vi "Add Calculate Channel_Formula_Formula.vi"(8 "error in (error out)":errorcluster, 9 "Formula Settings":T2, 10 "Calculated Channels Ref":refnum<k24>, 11 "SysDef Ref":T1) -> (0 "error out":errorcluster, 2 "Calculated Channels Ref Out":refnum<k24>)   [LabVIEW 2019, in "Simple SysDef API.lvlib"]
uses:
  <userlib>/SimpleSysDef/Simple SysDef API.lvlib
  NationalInstruments.VeriStand.SystemDefinitionAPI
  <userlib>/SimpleSysDef/_SubVIs/Add Calculate Channel_Formula_Settings.ctl
  <userlib>/SimpleSysDef/_SubVIs/System Definition Reference.ctl
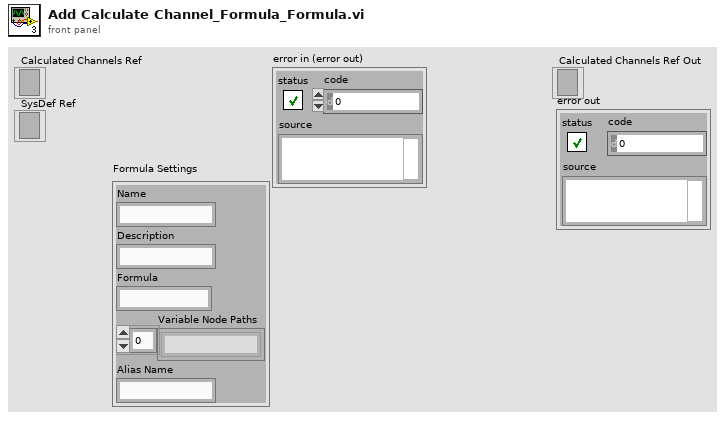
[diagram p1: front panel]
types:
  T1 = typedef "Simple SysDef API.lvlib/System Definition Reference.ctl" = refnum<k24>
  T2 = typedef "Simple SysDef API.lvlib/Add Calculate Channel_Formula_Settings.ctl" = cluster{"Name":string, "Description":string, "Formula":string, "Variable Node Paths":string[], "Alias Name":string}
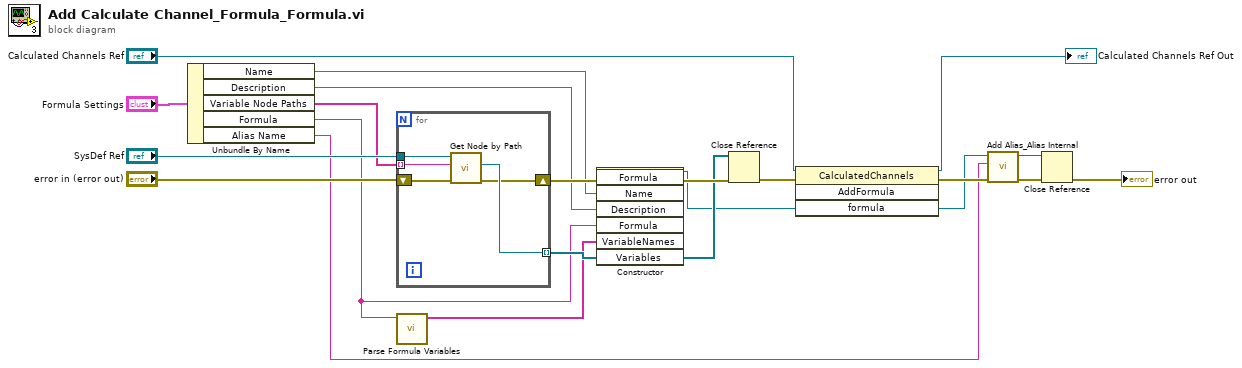
[diagram p0: block diagram]
diagram:
  n1 = Unbundle By Name("Formula Settings") -> ("Name"=w9:string, "Description"=w6:string, "Variable Node Paths"=w8:string[], "Formula"=w7:string, "Alias Name"=w1:string)
  n2 = for {
    tunnel: [w26] -> w15 mode=indexing
    shift-right: [w25] -> w11
    shift-left: "error in (error out)" -> [w24]
    tunnel: w8 -> [w23] mode=indexing
    tunnel: "SysDef Ref" -> [w22]
    n3 = call <userlib>:"Get Node by Path.vi"("error in (no error)"=w24, "System Definition Node Path"=w23, "SysDef Ref"=w22) -> ("error out"=w25:errorcluster, "Node Ref"=w26:refnum<k24>)  [unwired: 6 in, 1 out]
  }
  n4 = call <userlib>:"Parse Formula Variables.vi"("Formula"=w7) -> ("Variables"=w10:string[])  [unwired: 10 in]
  n5 = constructor class="Formula"(error in=w11, "Name"=w9, "Description"=w6, "Formula"=w7, "VariableNames"=w10, "Variables"=w15) -> (reference out=w3:refnum<k24>, error out=w14:errorcluster, "Variables"=w12:refnum<k24>[])  [unwired: 2 in, 5 out]
  n6 = Close Reference(reference=w12, error in (no error)=w14) -> (error out=w13:errorcluster)
  n7 = invoke class="CalculatedChannels" method="AddFormula"(reference="Calculated Channels Ref", error in=w13, "formula"=w3) -> (reference out=→"Calculated Channels Ref Out":refnum<k24>, error out=w5:errorcluster)  [unwired: 1 in, 2 out]
  n8 = call <userlib>:"Add Alias_Alias Internal.vi"("error in (no error)"=w5, "Name"=w1, "Base Node"=w3) -> ("error out"=w4:errorcluster, "Base Node out"=w2:refnum<k24>)  [unwired: 7 in]
  n9 = Close Reference(reference=w2, error in (no error)=w4) -> (error out=→"error out":errorcluster)
